vi "Channels to Block Conversions.vi"(7 "transfer configuration":T1, 9 "initial engine buffer offset":u64 format="%d bytes", 10 "initial string buffer offset":u64 format="%d bytes", 11 "Transfer Configuration":refnum<class "Transfer Configuration.lvclass">) -> (3 "Transfer conversion descriptors":T3[](array[typedef]) {"string offset" format="%d bytes"; "engine offset" format="%d bytes"})   [LabVIEW 2017, in "DSF Core.lvlib" / "Default Buffer Converter.lvclass"]
uses:
  Default Buffer Converter.lvclass
  Conversion Block.ctl
  Typedefs/DSF Data Type.ctl
  Classes/Configuration/Core/Transfer/Transfer Configuration.lvclass
  Configurations/Transfer Configuration.ctl
  Typedefs/DSF Byte Order.ctl
  Classes/Configuration/Core/Transfer/Transfer Configuration.lvclass/Transfer Configuration.ctl
  Classes/Framework/Framework.lvclass
  DSF Core.lvlib
  Configurations/Default Buffer Converter Transfer Configuration.lvclass
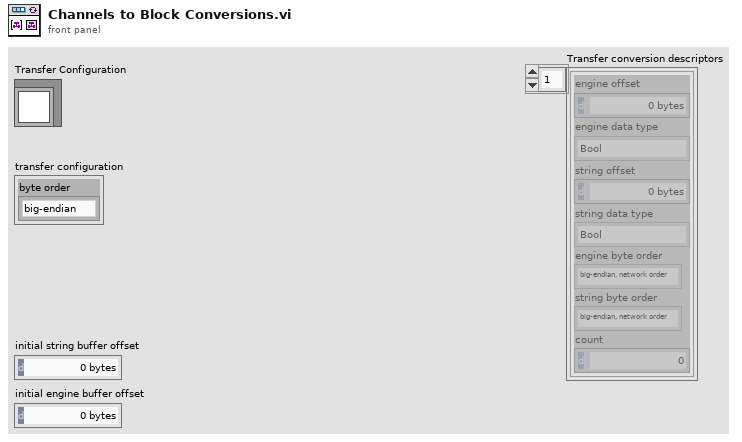
[diagram p1: front panel]
types:
  T1 = typedef "DSF Core.lvlib/Default Buffer Converter Transfer Configuration.lvclass/Transfer Configuration.ctl" = cluster{"byte order":T2}
  T2 = typedef "DSF Core.lvlib/DSF Byte Order.ctl" = enum8{"big-endian", "little-endian"}
  T3 = typedef "DSF Core.lvlib/Default Buffer Converter.lvclass/Conversion Block.ctl" = cluster{"engine offset":u64, "engine data type":T4, "string offset":u64, "string data type":T4, "engine byte order":enum16{"big-endian, network order", "native, host order", "little-endian"}, "string byte order":enum16{"big-endian, network order", "native, host order", "little-endian"}, "count":u64}
  T4 = typedef "DSF Core.lvlib/DSF Data Type.ctl" = enum8{"Bool", "SGL", "DBL", "I8", "I16", "I32", "I64", "U8", "U16", "U32", "U64"}
  T5 = enum16{"big-endian, network order", "native, host order", "little-endian"}
  T6 = typedef "DSF Core.lvlib/Transfer Configuration.lvclass/Channel Configuration.ctl" = cluster{"configuration":T7, "component settings":T8[]}
  T7 = typedef "DSF Core.lvlib/Channel Configuration.lvclass/Core Channel Configuration.ctl" = cluster{"name":string, "units":string, "engine data type":T4, "string data type":T4, "string offset":u64}
  T8 = typedef "DSF Core.lvlib/DSF Settings Info.ctl" = cluster{"component":string, "values":cluster{"key":string, "value":string}[]}
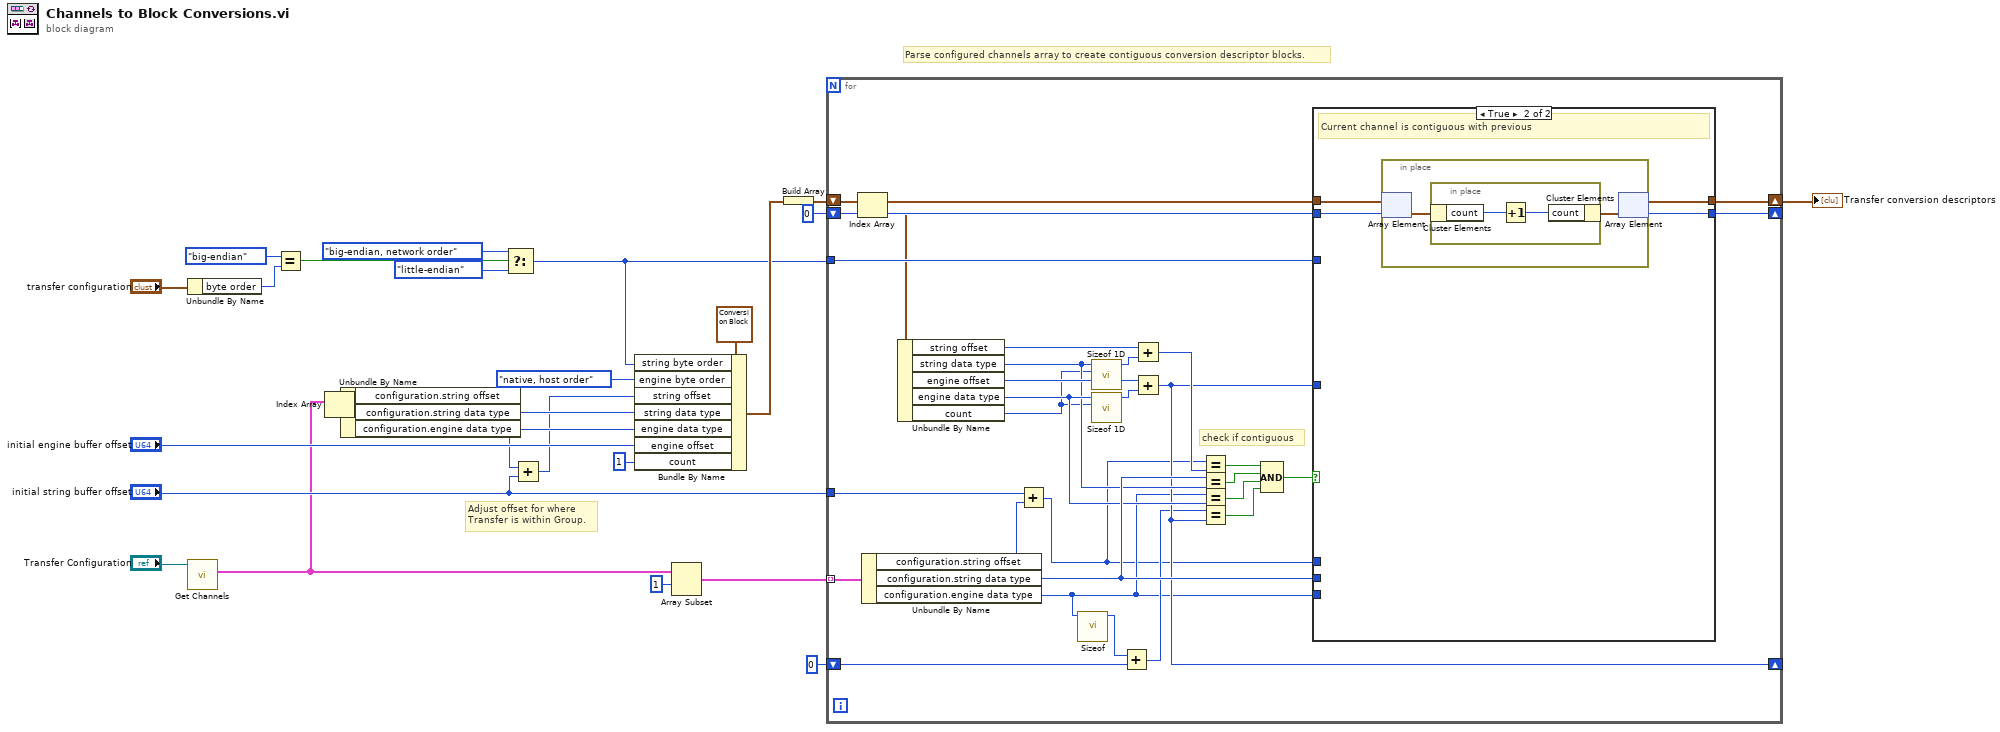
[diagram p0: block diagram]
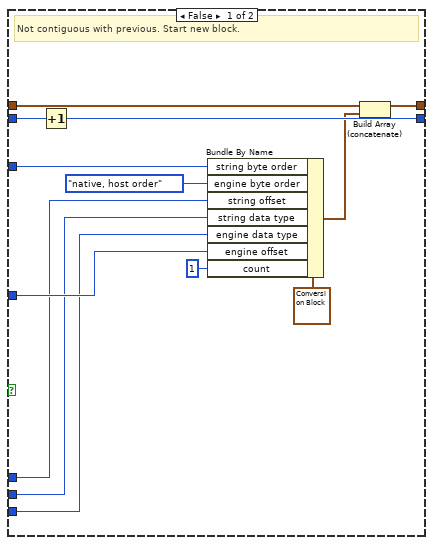
[diagram p2: hidden frame]
diagram:
  # "Adjust offset for where Transfer is within Group."
  # "Parse configured channels array to create contiguous conversion descriptor blocks."
  n1 = Unbundle By Name("transfer configuration") -> ("byte order"=w2:T2)
  n2 = call "Get Channels.vi"("Transfer Configuration in"="Transfer Configuration") -> ("channels"=w4:T6[])  [unwired: 8 in, 2 out]
  n3 = Equal?(x=DSF_Byte_Order."big-endian", y=w2) -> (x = y?=w26:bool)
  n4 = Index Array(array=w4) -> (element=w16:T6)  [unwired: 1 in]
  n5 = Unbundle By Name(w16) -> ("configuration.string offset"=w5:u64, "configuration.string data type"=w17:T4, "configuration.engine data type"=w12:T4)
  n6 = Select(t=T5."big-endian, network order" ("engine byte order"), s=w26, f=T5."little-endian" ("engine byte order")) -> (s? t:f=w8:T5)
  n7 = Add(x=w5, y="initial string buffer offset") -> (x+y=w6:u64)
  n8 = Bundle By Name(cluster=T3 {"engine offset"=0, "engine data type"=enum."Bool", "string offset"=0, "string data type"=enum."Bool", "engine byte order"=enum."big-endian, network order", "string byte order"=enum."big-endian, network order", "count"=0} ("conversion descriptor"), "string byte order"=w8, "engine byte order"=T5."native, host order", "string offset"=w6, "string data type"=w17, "engine data type"=w12, "engine offset"="initial engine buffer offset", "count"=u64 1) -> (w9:T3)
  n9 = Array Subset(array=w4, index=1) -> (w18:T6[])  [unwired: 1 in]
  n10 = Build Array(w9) -> (w13:T3[])
  n11 = for {
    tunnel: w18 -> [w55] mode=indexing
    tunnel: w8 -> [w54]
    shift-right: [w35] -> _
    shift-left: u64 0 -> [w32]
    shift-right: [w40] -> w15
    shift-left: w13 -> [w38]
    shift-right: [w39] -> _
    shift-left: 0 -> [w37]
    tunnel: "initial string buffer offset" -> [w29]
    # "check if contiguous"
    n12 = Index Array(array=w38, index=w37) -> (element=w36:T3)
    n13 = Unbundle By Name(w55) -> ("configuration.string offset"=w28:u64, "configuration.string data type"=w44:T4, "configuration.engine data type"=w30:T4)
    n14 = Unbundle By Name(w36) -> ("string offset"=w52:u64, "string data type"=w41:T4, "engine offset"=w42:u64, "engine data type"=w43:T4, "count"=w34:u64)
    n15 = Add(x=w29, y=w28) -> (x+y=w27:u64)
    n16 = call "Sizeof.vi"("data type"=w30) -> ("size in bytes"=w33:u64)  [unwired: 9 in, 1 out]
    n17 = call "Sizeof 1D.vi"("count"=w34, "data type"=w41) -> ("size in bytes"=w51:u64)  [unwired: 9 in]
    n18 = call "Sizeof 1D.vi"("count"=w34, "data type"=w43) -> ("size in bytes"=w53:u64)  [unwired: 9 in]
    n19 = Add(x=w33, y=w32) -> (x+y=w31:u64)
    n20 = Add(x=w52, y=w51) -> (x+y=w50:u64)
    n21 = Add(x=w42, y=w53) -> (x+y=w35:u64)
    n22 = Equal?(x=w27, y=w50) -> (x = y?=w49:bool)
    n23 = Equal?(x=w44, y=w41) -> (x = y?=w46:bool)
    n24 = Equal?(x=w30, y=w43) -> (x = y?=w47:bool)
    n25 = Equal?(x=w31, y=w35) -> (x = y?=w48:bool)
    n26 = Compound Arithmetic op=AND(w49, w46, w47, w48) -> (w45:bool)
    n27 = case shown="True" w45 {
      tunnel: w30 -> [w62 _]
      tunnel: w44 -> [w61 _]
      tunnel: w27 -> [w63 _]
      tunnel: w35 -> [w64 _]
      tunnel: w54 -> [w66 _]
      tunnel: w38 -> [w58 w72]
      tunnel: [w57 w69] -> w40
      tunnel: w37 -> [w60 w71]
      tunnel: [w59 w70] -> w39
      frame False {
        # "Not contiguous with previous. Start new block."
        n28 = Increment(x=w60) -> (x+1=w59:i32)
        n29 = Bundle By Name(cluster=T3 {"engine offset"=0, "engine data type"=enum."Bool", "string offset"=0, "string data type"=enum."Bool", "engine byte order"=enum."big-endian, network order", "string byte order"=enum."big-endian, network order", "count"=0} ("conversion descriptor"), "string byte order"=w66, "engine byte order"=T5."native, host order", "string offset"=w63, "string data type"=w61, "engine data type"=w62, "engine offset"=w64, "count"=u64 1) -> (w56:T3)
        n30 = Build Array (concatenate)(w58, w56) -> (w57:T3[])
      }
      frame True {
        # "Current channel is contiguous with previous"
        n31 = in-place {
          n32 = in-place-array #1(w72, w71) -> (w73:T3)
          n33 = in-place {
            n34 = in-place-cluster #2(w73) -> ("count"=w76:u64)
            n35 = Increment(x=w76) -> (x+1=w75:u64)
            n36 = in-place-cluster #2("count"=w75) -> (w74:T3)
          }
          n37 = in-place-array #1(w74) -> (w69:T3[], w70:i32)
        }
      }
    }
  }
  "Transfer conversion descriptors" <- w15
